vi "enumerateStaticDependencies.vi"(8 "error in (no error)":errorcluster, 11 "SMO.D":refnum<class "SMO.Configurable.lvclass">) -> (0 "error out":errorcluster, 2 "Static Dependencies":refnum<class "Dependency.lvclass">[](array[class]), 3 "SMO.D out":refnum<class "SMO.Configurable.lvclass">)   [LabVIEW 2013, in "SMO.Configurable.lvclass"]
uses:
  SMO.Configurable.lvclass
  src/Dependency/Dependency.lvclass
  src/SMO/SMO.lvclass
  SMO.B/SMO.B.lvclass
panel:
  # "For instructions on how to use the JKI State Machine Objects, examples and video tutorials, visit:\nhttp://jki.net/state-machine-objects/\n\nJKI State Machine Objects™\nhttp://jki.net/state-machine-objects/\nCopyright (C) 2005-2015, JKI <info@jki.net>\nALL RIGHTS RESERVED"
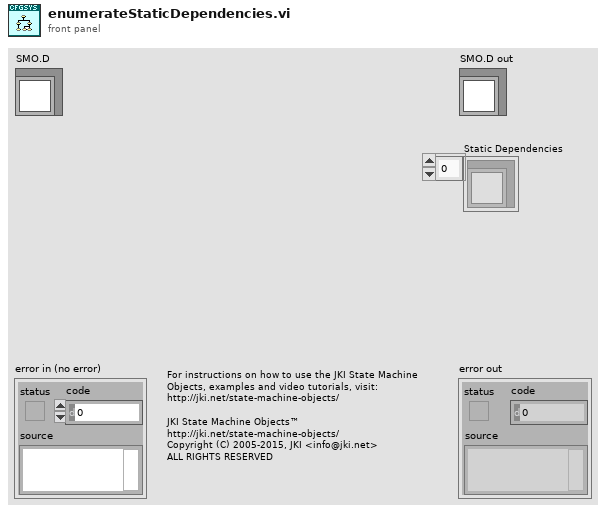
[diagram p1: front panel]
types:
  T1 = typedef "SMO.Configurable.lvclass/Config--cluster.ctl" = cluster{"timeout":i32, "run":bool}
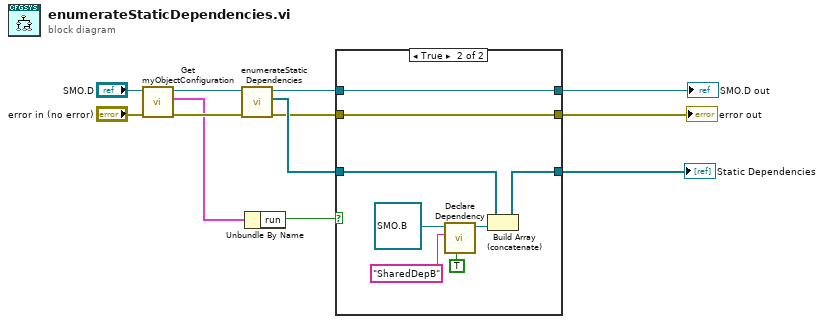
[diagram p0: block diagram]
diagram:
  n1 = call "Get myObjectConfiguration.vi"("error in (no error)"="error in (no error)", "SMO.Configurable in"="SMO.D") -> ("error out"=w8:errorcluster, "Config"=w6:T1, "SMO.Configurable out"=w10:refnum<class "SMO.Configurable.lvclass">)  [unwired: 7 in]
  n2 = call-parent "enumerateStaticDependencies.vi"("error in (no error)"=w8, "SMO"=w10) -> ("error out"=w3:errorcluster, "Static Dependencies"=w7:refnum<class "Dependency.lvclass">[], "SMO out"=w4:refnum<class "SMO.Configurable.lvclass">)  [unwired: 7 in]
  n3 = Unbundle By Name(w6) -> ("run"=w5:bool)
  n4 = case shown="True" w5 {
    tunnel: [w15 w18] -> w12
    tunnel: w7 -> [w15 w19]
    tunnel: w4 -> [w14 w17]
    tunnel: w3 -> [w13 w16]
    tunnel: [w14 w17] -> w1
    tunnel: [w13 w16] -> w2
    frame False {
    }
    frame True {
      n5 = call "Declare Dependency.vi"("Shared Resource (F)"=TRUE, "Name"="SharedDepB", "Type"=refnum<class "SMO.B.lvclass"> refnum ("SMO.B.lvclass")) -> ("Dependency out"=w21:refnum<class "Dependency.lvclass">)  [unwired: 7 in, 1 out]
      n6 = Build Array (concatenate)(w19, w21) -> (w18:refnum<class "Dependency.lvclass">[])
    }
  }
  "error out" <- w2
  "SMO.D out" <- w1
  "Static Dependencies" <- w12
